vi "datalogger_all_signals_v3.0.vi"() -> ()   [LabVIEW 2017]
uses:
  <vilib>/Utility/file.llb/Write Delimited Spreadsheet (string).vi
  <vilib>/NI/Modbus Library/API/Wrapper/Create TCP Master.vi
  <vilib>/NI/Modbus Library/API/Master/Modbus Master.lvclass
  <instrlib>/Agilent 34970/Agilent 34970.lvlib
  <vilib>/NI/Modbus Library/API/Wrapper/API Main.lvlib
panel:
  out "Time constant 2":i32
  out "Time constant":i32
  in  "Tab Control":T1(tab)
  out "Indicator":bool
  in  "Touch the button to refresh":bool
  in  "Power on/off":u16(ring) items=["Power off", "Powe on"]
  in  "Mode selector":u16(ring) items=["Conditioning", "Activation"]
  out "Mode status":string
  out "Controller output 3 (V)":u16[](array[numeric])
  out "Controller outpu 2 (V)":u16[](array[numeric])
  out "Controller output 1 (V)":u16[](array[numeric])
  in  "Stop test":bool
  out "Controller temperature (Cº)":dbl[](array[numeric])
  out "Coil tempe (Cº)":dbl[](array[numeric])
  out "PT100 temp (Cº)":ext[](array[numeric])
  out "sampling time (ms)":u32
  out "Power consuption (W)":dbl[](array[numeric]) format="%.2f"
  in  "Datalogger_current\nGPIB1":refnum<visa-resource-name>="GPIB0::9::INSTR"
  in  "Datalogger_all_signals\nGPIB0":refnum<visa-resource-name>="GPIB0::9::INSTR"
  in  "Test type":u16(ring) items=["Final", "INITIAL", "PASSIVE", "ACTIVE"]
  in  "Axis orientation":u16(ring) items=["+x", "-x", "+y", "-y", "+z", "-z", "Reference Test"]
  out "minutos":u32
  out "segundos":u32
  out "Heating resistor 1":cluster{dbl[], dbl[]}[](graph)
  out "Heating resistor 1  DC voltage (v)":dbl[](array[numeric]) format="%.6f"
  out "Termocouple out1":dbl[](array[numeric])
  out "Heating resistor 1 P out (W)":dbl[](array[numeric])
  out "Heat resistor 1 resistance":dbl[](array[numeric]) format="%.2f"
  out "Heating resistor 2  DC voltage (v)":dbl[](array[numeric]) format="%.6f"
  out "Heating resistor 2 P out (W)":dbl[](array[numeric])
  out "Termocouple out2":dbl[](array[numeric])
  out "Heating resistor 2":cluster{dbl[], dbl[]}[](graph)
  out "Heat resistor 2 resistance":dbl[](array[numeric]) format="%.2f"
  out "Heating resistor 3  DC voltage (v)":dbl[](array[numeric]) format="%.6f"
  out "Heating resistor 3 P out (W)":dbl[](array[numeric])
  out "Termocouple out3":dbl[](array[numeric])
  out "Heating resistor 3":cluster{dbl[], dbl[]}[](graph)
  out "Heat resistor 3 resistance":dbl[](array[numeric]) format="%.2f"
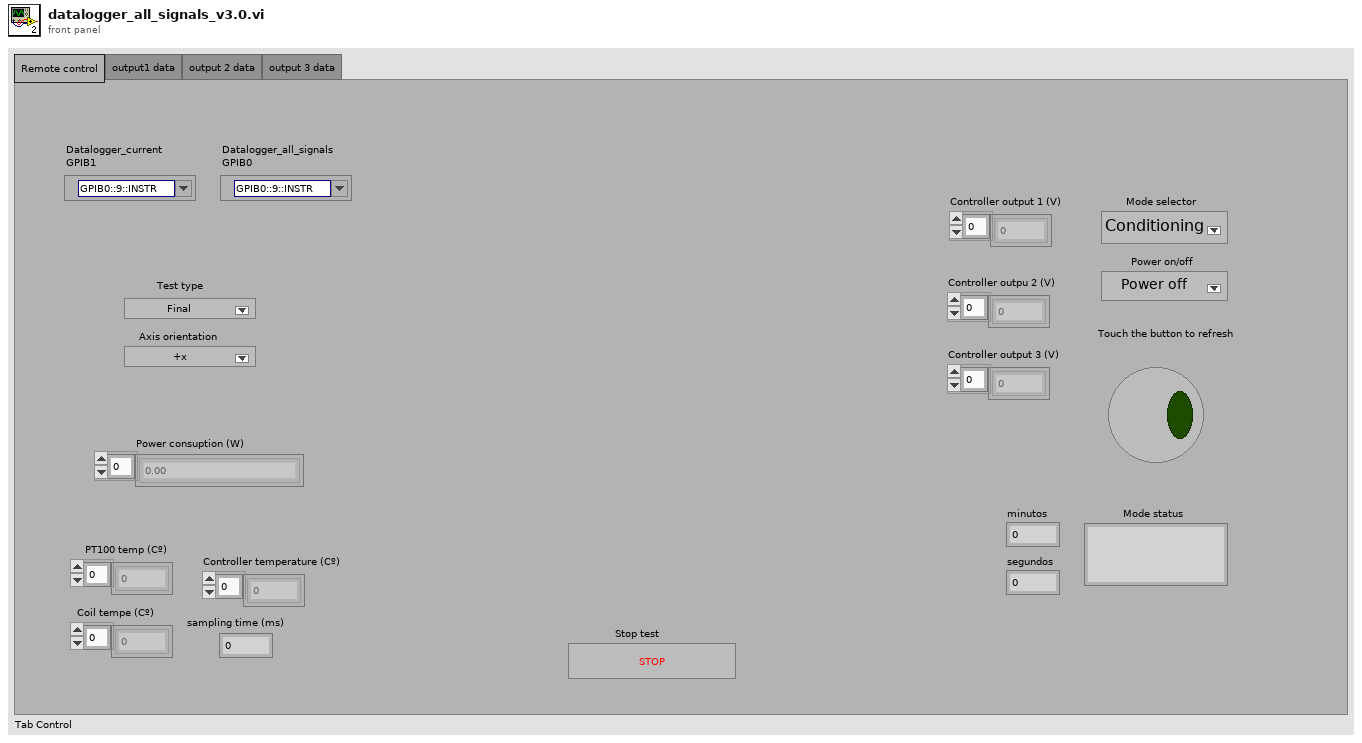
[diagram p1: front panel]
types:
  T1 = enum32{"Remote control", "output1 data", "output 2 data", "output 3 data"}
  T2 = enum16{"100 Ohm", "1 kOhm", "10 kOhm", "100 kOhm", "1 MOhm", "10 MOhm", "100 MOhm", "Auto", "Minimum", "Maximum"}
  T3 = enum16{"4 1/2", "5 1/2", "6 1/2", "Least", "Highest", "Default"}
  T4 = enum16{"100 mV", "1 V", "10 V", "100 V", "300 V", "Auto", "Minimum", "Maximum"}
  T5 = enum16{"B", "E", "J", "K", "N", "R", "S", "T", "Default (Last)"}
  T6 = enum16{"Thermocouple", "Thermistor", "RTD", "4-Wire RTD", "Default (Last)"}
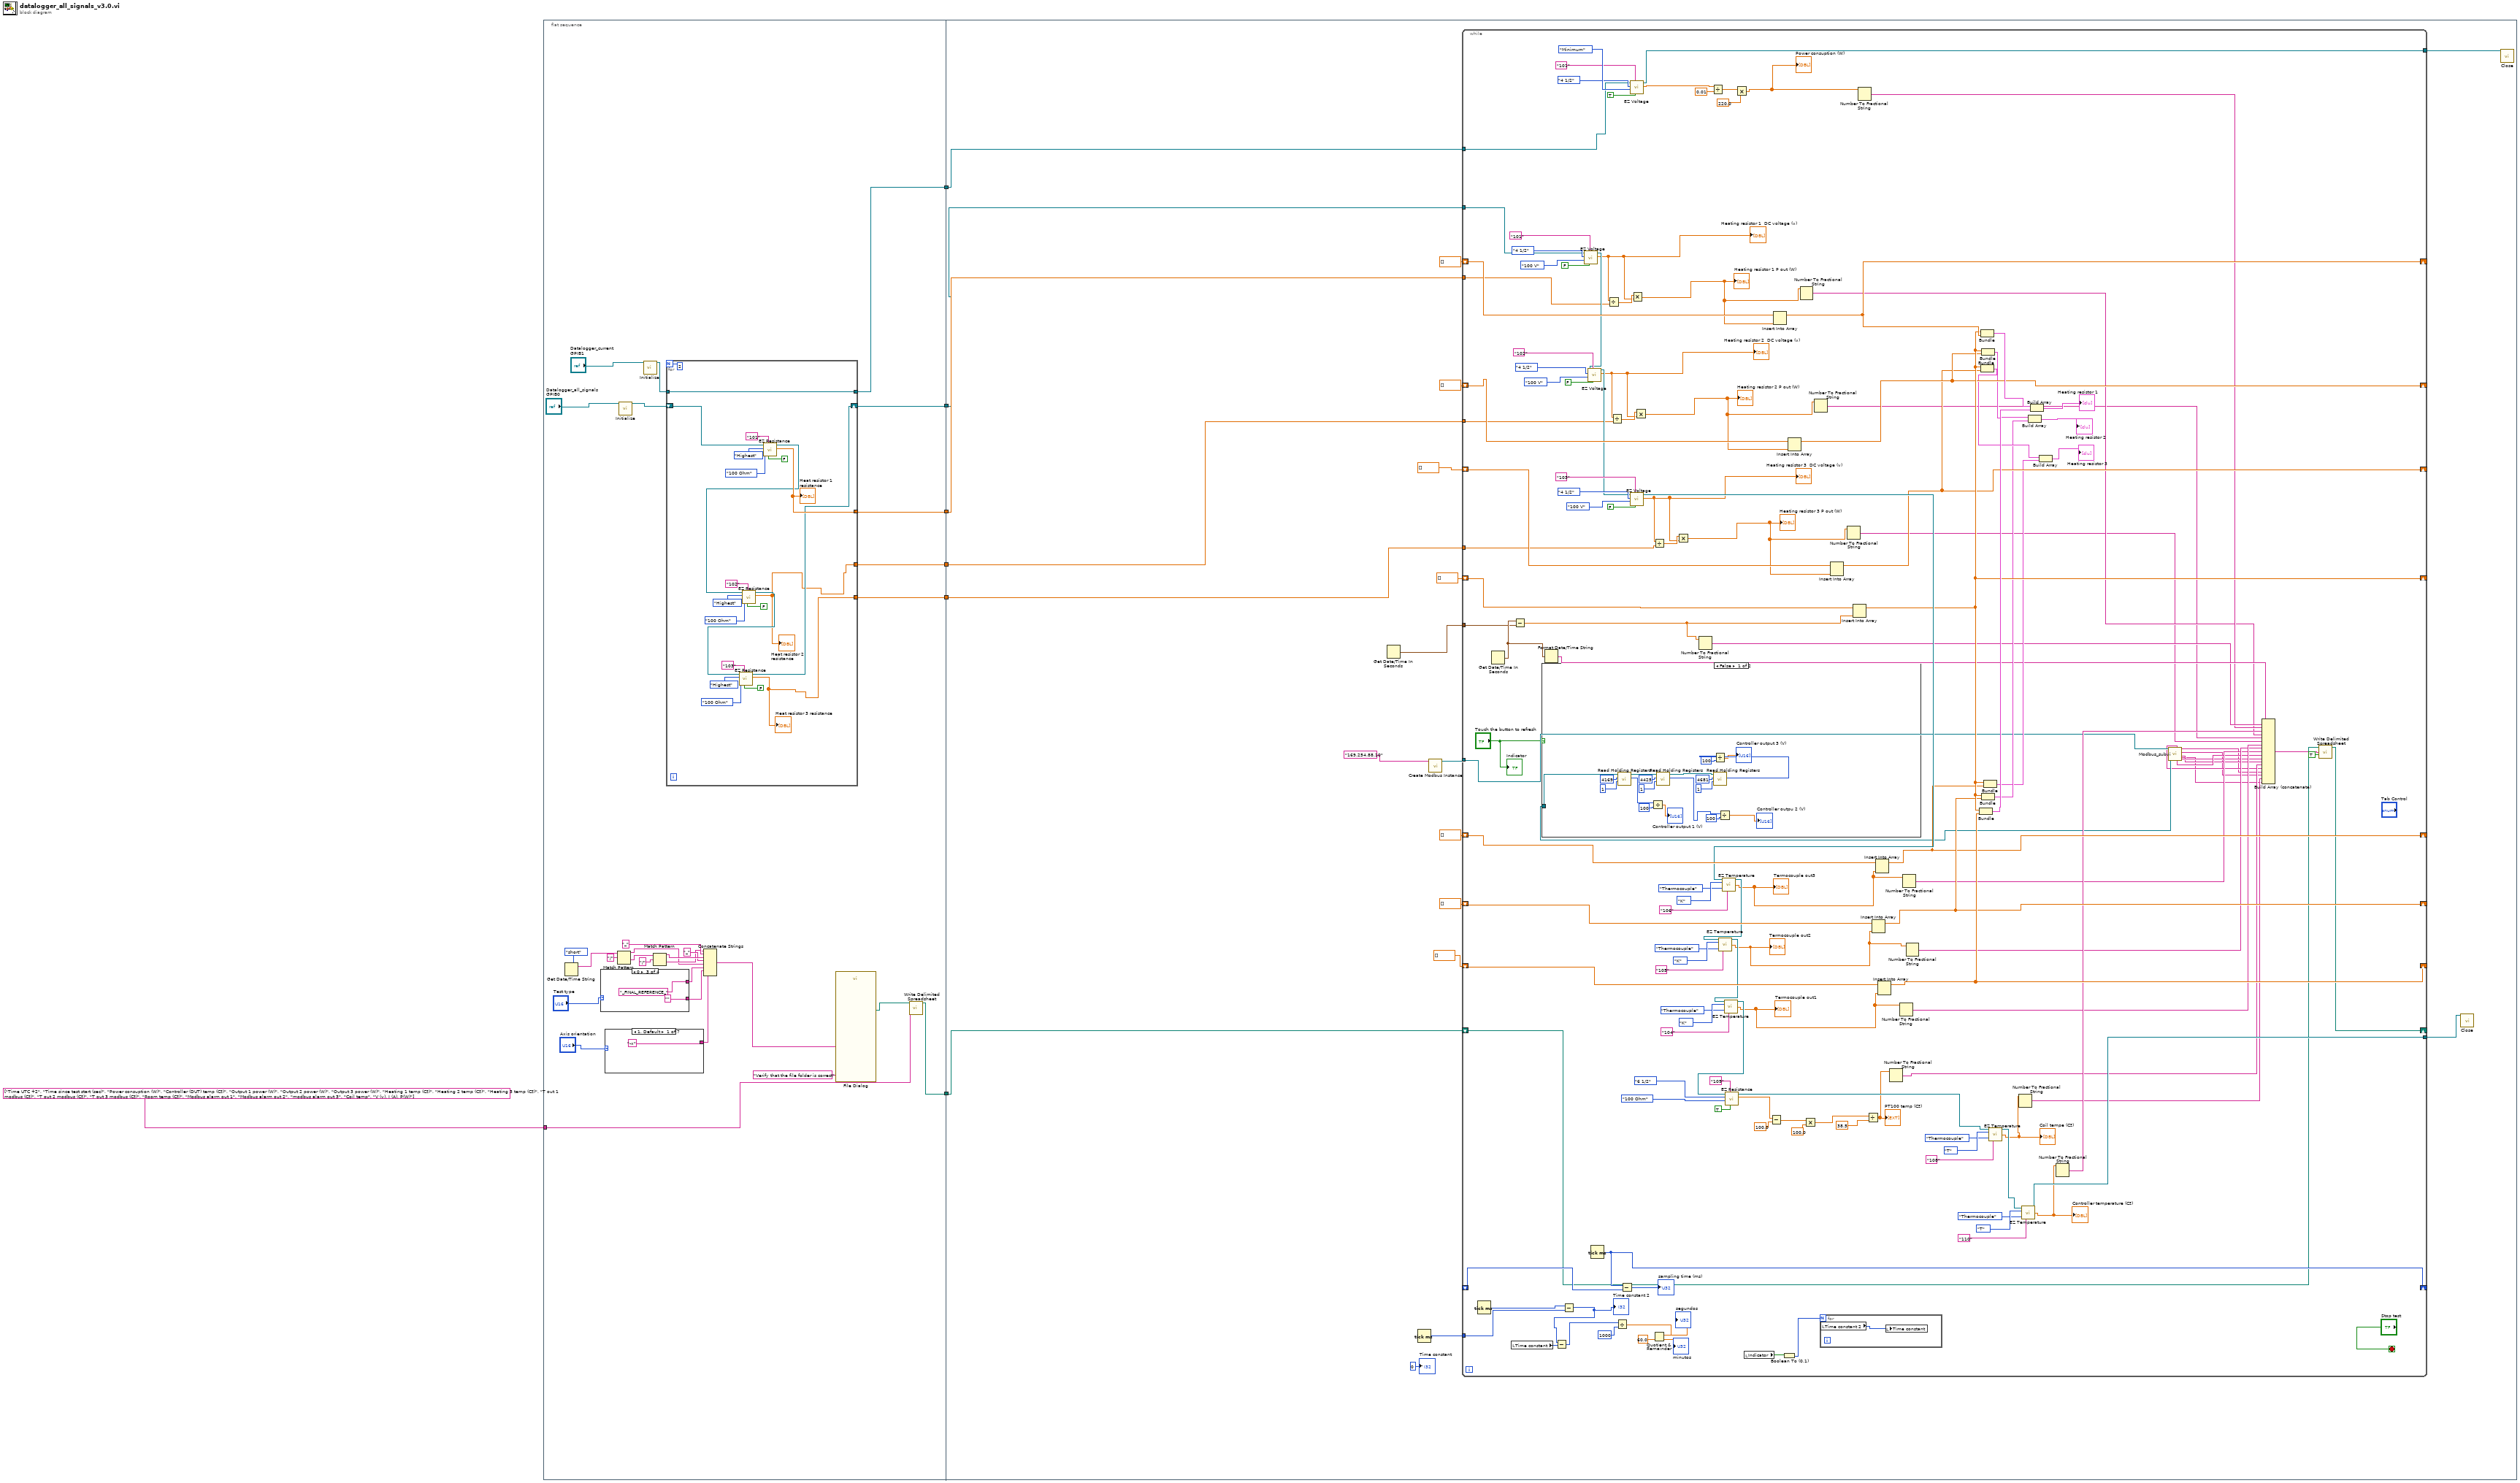
[diagram p0: block diagram]
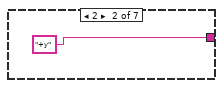
[diagram p2: hidden frame]
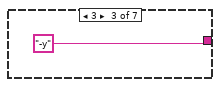
[diagram p3: hidden frame]
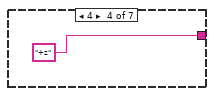
[diagram p4: hidden frame]
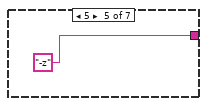
[diagram p5: hidden frame]
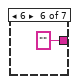
[diagram p6: hidden frame]
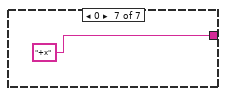
[diagram p7: hidden frame]
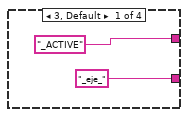
[diagram p8: hidden frame]
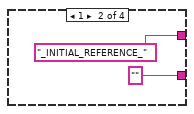
[diagram p9: hidden frame]
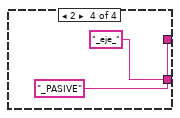
[diagram p10: hidden frame]
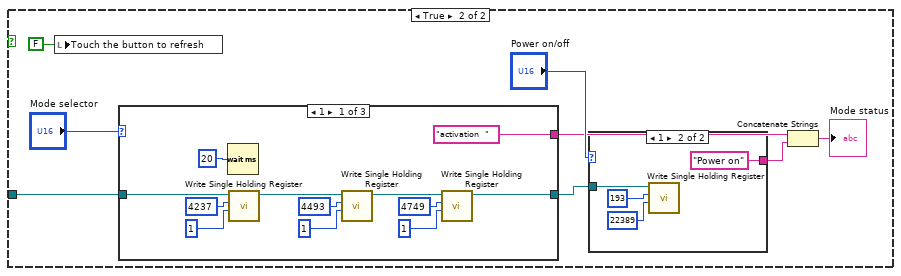
[diagram p11: hidden frame]
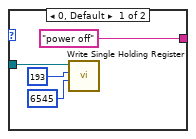
[diagram p12: hidden frame]
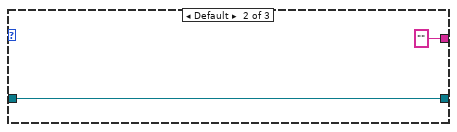
[diagram p13: hidden frame]
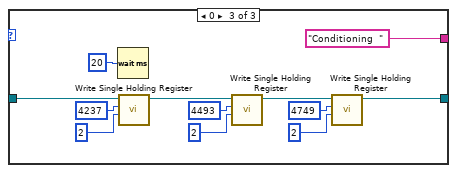
[diagram p14: hidden frame]
diagram:
  n1 = flat-sequence {
    tunnel: string[] ["Time UTC +2", "Time since test start (sec)", "Power consuption (W)", "Controller (DUT) temp (Cº)", "Output 1 power (W)", "Output 2 power (W)", "Output 3 power (W)", "Heating 1 temp (Cº)", "Heating 2 temp (Cº)", "Heating 3 temp (Cº)", "T out 1 modbus (Cº)", "T out 2 modbus (Cº)", "T out 3 modbus (Cº)", "Room temp (Cº)", "Modbus alarm out 1", "Modbus alarm out 2", "modbus alarm out 3", "Coil temp", "V (v), I (A), P(W)"] ("element") -> [w30]
    tunnel: [w34] -> w6
    tunnel: [w33] -> w5
    tunnel: [w32] -> w4
    tunnel: [w29] -> w3
    tunnel: [w28] -> w2
    tunnel: [w25] -> w1
    tunnel: w6 -> [w89]
    tunnel: w5 -> [w82]
    tunnel: w4 -> [w81]
    tunnel: w3 -> [w80]
    tunnel: w2 -> [w79]
    tunnel: w1 -> [w78]
    frame #0 {
      n2 = Get Date/Time String(date format (0)=enum16{"short", "long", "abbreviated"}."short") -> (date string=w19:string)  [unwired: 2 in, 1 out]
      n3 = case shown="0" "Test type" {
        tunnel: ["_ACTIVE" "_INITIAL_REFERENCE_" "_FINAL_REFERENCE_" "_PASIVE"] -> w23
        tunnel: ["_eje_" ("string") "" ("string") "" ("string") "_eje_" ("string")] -> w12
        frame 3, Default {
        }
        frame 1 {
        }
        frame 0 {
        }
        frame 2 {
        }
      }
      n4 = case shown="1, Default" "Axis orientation" {
        tunnel: ["-x" "+y" "-y" "+z" "-z" "" "+x"] -> w20
        frame 1, Default {
        }
        frame 2 {
        }
        frame 3 {
        }
        frame 4 {
        }
        frame 5 {
        }
        frame 6 {
        }
        frame 0 {
        }
      }
      n5 = Match Pattern(string=w19, regular expression="/") -> (before substring=w9:string, after substring=w16:string)  [unwired: 1 in, 2 out]
      n6 = call <instrlib>:"Initialize.vi"("VISA Resource Name"="Datalogger_all_signals\nGPIB0") -> ("VISA Resource Name Out"=w36:refnum<visa-resource-name>)  [unwired: 13 in, 1 out]
      n7 = call <instrlib>:"Initialize.vi"("VISA Resource Name"="Datalogger_current\nGPIB1") -> ("VISA Resource Name Out"=w26:refnum<visa-resource-name>)  [unwired: 13 in, 1 out]
      n8 = Match Pattern(string=w16, regular expression="/") -> (before substring=w14:string, after substring=w11:string)  [unwired: 1 in, 2 out]
      n9 = for {
        N: 2 -> [_]
        tunnel: [w67] -> w34
        shift-right: [w56] -> w28
        shift-left: w36 -> [w69]
        tunnel: [w55] -> w33
        tunnel: [w54] -> w32
        tunnel: w26 -> [w53]
        tunnel: [w53] -> w25
        n10 = call <instrlib>:"EZ Resistance.vi"("2w/4w (F:2w)"=FALSE, "Scan List (empty)"="101", "Range (7:Auto)"=T2."100 Ohm", "Resolution (5:Default)"=T3."Highest", "VISA Resource Name"=w69) -> ("Output Array"=w67:dbl[], "VISA Resource Name Out"=w58:refnum<visa-resource-name>)  [unwired: 4 in, 1 out]
        "Heat resistor 1 resistance" <- w67
        n11 = call <instrlib>:"EZ Resistance.vi"("2w/4w (F:2w)"=FALSE, "Scan List (empty)"="102", "Range (7:Auto)"=T2."100 Ohm", "Resolution (5:Default)"=T3."Highest", "VISA Resource Name"=w58) -> ("Output Array"=w55:dbl[], "VISA Resource Name Out"=w57:refnum<visa-resource-name>)  [unwired: 4 in, 1 out]
        "Heat resistor 2 resistance" <- w55
        n12 = call <instrlib>:"EZ Resistance.vi"("2w/4w (F:2w)"=FALSE, "Scan List (empty)"="103", "Range (7:Auto)"=T2."100 Ohm", "Resolution (5:Default)"=T3."Highest", "VISA Resource Name"=w57) -> ("Output Array"=w54:dbl[], "VISA Resource Name Out"=w56:refnum<visa-resource-name>)  [unwired: 4 in, 1 out]
        "Heat resistor 3 resistance" <- w54
      }
      n13 = Concatenate Strings(w11, "_" ("string"), w14, "_" ("string"), w9, w23, w12, w20) -> (w10:string)
      n14 = call "File Dialog"("prompt"="Verify that the file folder is correct", "default name"=w10) -> ("selected path"=w31:path)  [unwired: 10 in, 3 out]
      n15 = call-poly <vilib>:"Write Delimited Spreadsheet.vi"("file path (dialog if empty)"=w31, "1D data"=w30) -> ("new file path (Not A Path if cancelled)"=w29:path)  [unwired: 12 in, 1 out]
    }
    frame #1 {
      n16 = Get Date/Time In Seconds() -> (seconds since 1Jan1904=w75:timestamp)
      n17 = Tick Count (ms)() -> (millisecond timer value=w74:u32)
      n18 = call-poly <vilib>:"Create Modbus Instance.vi"("address"="169.254.88.10") -> ("TCP master instance"=w92:refnum<class "Modbus Master.lvclass">)  [unwired: 9 in, 1 out]
      n19 = while {
        shift-right: [w231] -> _
        shift-left: _ -> [w230]
        tunnel: w89 -> [w175]
        shift-right: [w206] -> _
        shift-left: dbl[] [] -> [w208]
        shift-right: [w174] -> _
        shift-left: dbl[] [] -> [w207]
        shift-right: [w203] -> _
        shift-left: dbl[] [] -> [w205]
        shift-right: [w171] -> _
        shift-left: dbl[] [] -> [w195]
        shift-right: [w166] -> _
        shift-left: dbl[] [] -> [w189]
        shift-right: [w173] -> _
        shift-left: dbl[] [] -> [w185]
        shift-right: [w172] -> _
        shift-left: dbl[] [] -> [w180]
        tunnel: [w155] -> w90
        tunnel: w82 -> [w154]
        tunnel: w81 -> [w153]
        shift-right: [w137] -> _
        shift-left: w80 -> [w138]
        tunnel: w79 -> [w134]
        tunnel: [w133] -> w91
        tunnel: w78 -> [w132]
        tunnel: w92 -> [w118]
        tunnel: w75 -> [w108]
        tunnel: w74 -> [w100]
        stop <- "Stop test" stop-if-true
        n20 = Tick Count (ms)() -> (millisecond timer value=w101:u32)
        n21 = Get Date/Time In Seconds() -> (seconds since 1Jan1904=w152:timestamp)
        n22 = local read "Time constant"() -> (w99:i32)
        n23 = Subtract(x=w152, y=w108) -> (x-y=w128:dbl)
        n24 = Format Date/Time String(seconds (now)=w152) -> (date/time string=w151:string)  [unwired: 2 in]
        n25 = Subtract(x=w101, y=w100) -> (x-y=w94:u32)
        "Time constant 2" <- w94
        n26 = Subtract(x=w94, y=w99) -> (x-y=w98:u32)
        n27 = call <instrlib>:"EZ Voltage.vi"("AC/DC (F:DC)"=FALSE, "Scan List (empty)"="101", "Range (5:Auto)"=T4."100 V", "Resolution (5:Default)"=T3."4 1/2", "VISA Resource Name"=w134) -> ("Output Array"=w150:dbl[], "VISA Resource Name Out"=w178:refnum<visa-resource-name>)  [unwired: 4 in, 1 out]
        "Heating resistor 1  DC voltage (v)" <- w150
        n28 = call <instrlib>:"EZ Voltage.vi"("AC/DC (F:DC)"=FALSE, "Scan List (empty)"="102", "Range (5:Auto)"=T4."100 V", "Resolution (5:Default)"=T3."4 1/2", "VISA Resource Name"=w178) -> ("Output Array"=w148:dbl[], "VISA Resource Name Out"=w177:refnum<visa-resource-name>)  [unwired: 4 in, 1 out]
        "Heating resistor 2  DC voltage (v)" <- w148
        n29 = Tick Count (ms)() -> (millisecond timer value=w231:u32)
        n30 = Divide(x=w150, y=w175) -> (x/y=w209:dbl[])
        n31 = Divide(x=w148, y=w154) -> (x/y=w196:dbl[])
        n32 = Divide(x=w98, y=u32 1000) -> (x/y=w104:dbl)
        n33 = Subtract(x=w231, y=w230) -> (x-y=→"sampling time (ms)":u32)
        n34 = call <instrlib>:"EZ Voltage.vi"("AC/DC (F:DC)"=TRUE, "Scan List (empty)"="101", "Range (5:Auto)"=T4."Minimum", "Resolution (5:Default)"=T3."4 1/2", "VISA Resource Name"=w132) -> ("Output Array"=w232:dbl[], "VISA Resource Name Out"=w133:refnum<visa-resource-name>)  [unwired: 4 in, 1 out]
        n35 = call <instrlib>:"EZ Voltage.vi"("AC/DC (F:DC)"=FALSE, "Scan List (empty)"="103", "Range (5:Auto)"=T4."100 V", "Resolution (5:Default)"=T3."4 1/2", "VISA Resource Name"=w177) -> ("Output Array"=w146:dbl[], "VISA Resource Name Out"=w176:refnum<visa-resource-name>)  [unwired: 4 in, 1 out]
        "Heating resistor 3  DC voltage (v)" <- w146
        n36 = Multiply(x=w209, y=w150) -> (x*y=w149:dbl[])
        "Heating resistor 1 P out (W)" <- w149
        n37 = Multiply(x=w196, y=w148) -> (x*y=w147:dbl[])
        "Heating resistor 2 P out (W)" <- w147
        n38 = Quotient & Remainder(x=w104, y=60.0) -> (x-y*floor(x/y)=→"segundos":dbl, floor(x/y)=→"minutos":dbl)
        n39 = Divide(x=w146, y=w153) -> (x/y=w190:dbl[])
        n40 = Multiply(x=w190, y=w146) -> (x*y=w145:dbl[])
        "Heating resistor 3 P out (W)" <- w145
        n41 = Number To Fractional String(number=w128) -> (F-format string=w127:string)  [unwired: 3 in]
        n42 = Divide(x=w232, y=0.01) -> (x/y=w131:dbl[])
        n43 = call <instrlib>:"EZ Temperature.vi"("VISA Resource Name"=w176, "Scan List (empty)"="106" ("Channel List"), "Thermocouple Type (8:Def-Last)"=T5."K", "Transducer Type (4:Def-Last)"=T6."Thermocouple") -> ("VISA Resource Name Out"=w179:refnum<visa-resource-name>, "Output Array"=w142:dbl[])  [unwired: 9 in, 1 out]
        "Termocouple out3" <- w142
        n44 = call <instrlib>:"EZ Temperature.vi"("VISA Resource Name"=w179, "Scan List (empty)"="105" ("Channel List"), "Thermocouple Type (8:Def-Last)"=T5."K", "Transducer Type (4:Def-Last)"=T6."Thermocouple") -> ("VISA Resource Name Out"=w184:refnum<visa-resource-name>, "Output Array"=w143:dbl[])  [unwired: 9 in, 1 out]
        "Termocouple out2" <- w143
        n45 = call <instrlib>:"EZ Temperature.vi"("VISA Resource Name"=w184, "Scan List (empty)"="104" ("Channel List"), "Thermocouple Type (8:Def-Last)"=T5."K", "Transducer Type (4:Def-Last)"=T6."Thermocouple") -> ("VISA Resource Name Out"=w210:refnum<visa-resource-name>, "Output Array"=w144:dbl[])  [unwired: 9 in, 1 out]
        "Termocouple out1" <- w144
        n46 = call <instrlib>:"EZ Resistance.vi"("2w/4w (F:2w)"=TRUE, "Scan List (empty)"="109", "Range (7:Auto)"=T2."100 Ohm", "Resolution (5:Default)"=T3."6 1/2", "VISA Resource Name"=w210) -> ("Output Array"=w213:dbl[], "VISA Resource Name Out"=w160:refnum<visa-resource-name>)  [unwired: 4 in, 1 out]
        n47 = Multiply(x=w131, y=220.0) -> (x*y=w129:dbl[])
        "Power consuption (W)" <- w129
        n48 = local read "Indicator"() -> (w96:bool)
        n49 = Subtract(x=w213, y=100.0) -> (x-y=w211:dbl[])
        n50 = Insert Into Array(array=w205, new element=w149) -> (w203:dbl[])  [unwired: 1 in]
        n51 = Boolean To (0,1)(Boolean=w96) -> (0, 1=w95:i16)
        n52 = Insert Into Array(array=w195, new element=w147) -> (w171:dbl[])  [unwired: 1 in]
        n53 = Number To Fractional String(number=w149) -> (F-format string=w124:string[])  [unwired: 3 in]
        n54 = Multiply(x=w211, y=100.0) -> (x*y=w215:ext[])
        n55 = Number To Fractional String(number=w147) -> (F-format string=w123:string[])  [unwired: 3 in]
        n56 = for {
          N: w95 -> [_]
          n57 = local read "Time constant 2"() -> (w237:i32)
          n58 = local write "Time constant"(w237) -> ()
        }
        n59 = Insert Into Array(array=w189, new element=w145) -> (w166:dbl[])  [unwired: 1 in]
        n60 = Number To Fractional String(number=w145) -> (F-format string=w122:string[])  [unwired: 3 in]
        n61 = Insert Into Array(array=w207, new element=w128) -> (w174:dbl[])  [unwired: 1 in]
        n62 = Number To Fractional String(number=w129) -> (F-format string=w126:string[])  [unwired: 3 in]
        n63 = Divide(x=w215, y=38.5) -> (x/y=w141:ext[])
        "PT100 temp (Cº)" <- w141
        n64 = Insert Into Array(array=w185, new element=w143) -> (w173:dbl[])  [unwired: 1 in]
        n65 = Insert Into Array(array=w180, new element=w142) -> (w172:dbl[])  [unwired: 1 in]
        n66 = Insert Into Array(array=w208, new element=w144) -> (w206:dbl[])  [unwired: 1 in]
        n67 = Number To Fractional String(number=w141) -> (F-format string=w113:string[])  [unwired: 3 in]
        n68 = Number To Fractional String(number=w144) -> (F-format string=w121:string[])  [unwired: 3 in]
        n69 = Number To Fractional String(number=w142) -> (F-format string=w119:string[])  [unwired: 3 in]
        n70 = Number To Fractional String(number=w143) -> (F-format string=w120:string[])  [unwired: 3 in]
        n71 = Bundle(w174, w206) -> (w204:cluster{dbl[], dbl[]})  [unwired: 1 in]
        n72 = Bundle(w174, w203) -> (w202:cluster{dbl[], dbl[]})  [unwired: 1 in]
        n73 = Bundle(w174, w166) -> (w167:cluster{dbl[], dbl[]})  [unwired: 1 in]
        n74 = Bundle(w174, w171) -> (w168:cluster{dbl[], dbl[]})  [unwired: 1 in]
        n75 = Bundle(w174, w173) -> (w165:cluster{dbl[], dbl[]})  [unwired: 1 in]
        n76 = Bundle(w174, w172) -> (w164:cluster{dbl[], dbl[]})  [unwired: 1 in]
        n77 = call <instrlib>:"EZ Temperature.vi"("VISA Resource Name"=w160, "Scan List (empty)"="108" ("Channel List"), "Thermocouple Type (8:Def-Last)"=T5."T", "Transducer Type (4:Def-Last)"=T6."Thermocouple") -> ("VISA Resource Name Out"=w156:refnum<visa-resource-name>, "Output Array"=w140:dbl[])  [unwired: 9 in, 1 out]
        "Coil tempe (Cº)" <- w140
        n78 = Number To Fractional String(number=w140) -> (F-format string=w109:string[])  [unwired: 3 in]
        n79 = call <instrlib>:"EZ Temperature.vi"("VISA Resource Name"=w156, "Scan List (empty)"="110" ("Channel List"), "Thermocouple Type (8:Def-Last)"=T5."T", "Transducer Type (4:Def-Last)"=T6."Thermocouple") -> ("VISA Resource Name Out"=w155:refnum<visa-resource-name>, "Output Array"=w139:dbl[])  [unwired: 9 in, 1 out]
        "Controller temperature (Cº)" <- w139
        n80 = Build Array(w168, w165) -> (→"Heating resistor 2":cluster{dbl[], dbl[]}[])
        n81 = Build Array(w202, w204) -> (→"Heating resistor 1":cluster{dbl[], dbl[]}[])
        n82 = Build Array(w167, w164) -> (→"Heating resistor 3":cluster{dbl[], dbl[]}[])
        n83 = Number To Fractional String(number=w139) -> (F-format string=w125:string[])  [unwired: 3 in]
        n84 = call "Modbus_subvi.vi"("Modbus master in"=w118) -> ("Output 2 temp alarm"=w115:string, "Output 3 temp alarm"=w114:string, "Controller output 3 alarm"=w110:string, "Controller output 2 alarm"=w111:string, "Output 1 temp alarm"=w116:string, "Controller output 1 alarm"=w112:string, "Variables voltage"=w93:string, "Modbus master out"=w117:refnum<class "Modbus Master.lvclass">)  [unwired: 3 in]
        n85 = case shown="False" "Touch the button to refresh" {
          tunnel: w117 -> [w253 w256]
          frame False {
            n86 = call-dynamic "Read Holding Registers.vi"("number of inputs"=u16 1, "starting address"=u32 4169, "Modbus master in"=w253) -> ("register values"=w246:u16[], "Modbus master out"=w248:refnum<class "Modbus Master.lvclass">)  [unwired: 6 in, 1 out]
            n87 = Divide(x=w246, y=u16 100) -> (x/y=→"Controller output 1 (V)":dbl[])
            n88 = call-dynamic "Read Holding Registers.vi"("number of inputs"=u16 1, "starting address"=u32 4425, "Modbus master in"=w248) -> ("register values"=w241:u16[], "Modbus master out"=w247:refnum<class "Modbus Master.lvclass">)  [unwired: 6 in, 1 out]
            n89 = call-dynamic "Read Holding Registers.vi"("number of inputs"=u16 1, "starting address"=u32 4681, "Modbus master in"=w247) -> ("register values"=w240:u16[])  [unwired: 6 in, 2 out]
            n90 = Divide(x=w240, y=u16 100) -> (x/y=→"Controller output 3 (V)":dbl[])
            n91 = Divide(x=w241, y=u16 100) -> (x/y=→"Controller outpu 2 (V)":dbl[])
          }
          frame True {
            n92 = local write "Touch the button to refresh"(FALSE ("Boolean")) -> ()
            n93 = case shown="1" "Mode selector" {
              tunnel: w256 -> [w275 w285 w289]
              tunnel: [w274 w285 w288] -> w262
              tunnel: ["activation  " ("Mode") "" ("Mode") "Conditioning  " ("Mode")] -> w259
              frame 1 {
                n94 = Wait (ms)(milliseconds to wait=u32 20) -> ()  [unwired: 1 out]
                n95 = call-dynamic "Write Single Holding Register.vi"("register to write"=u16 1 ("register to write 2"), "address"=u16 4237, "Modbus master in"=w275) -> ("Modbus master out"=w277:refnum<class "Modbus Master.lvclass">)  [unwired: 7 in, 1 out]
                n96 = call-dynamic "Write Single Holding Register.vi"("register to write"=u16 1 ("register to write 2"), "address"=u16 4493, "Modbus master in"=w277) -> ("Modbus master out"=w276:refnum<class "Modbus Master.lvclass">)  [unwired: 7 in, 1 out]
                n97 = call-dynamic "Write Single Holding Register.vi"("register to write"=u16 1 ("register to write 2"), "address"=u16 4749, "Modbus master in"=w276) -> ("Modbus master out"=w274:refnum<class "Modbus Master.lvclass">)  [unwired: 7 in, 1 out]
              }
              frame Default {
              }
              frame 0 {
                n98 = Wait (ms)(milliseconds to wait=u32 20) -> ()  [unwired: 1 out]
                n99 = call-dynamic "Write Single Holding Register.vi"("register to write"=u16 2 ("register to write 2"), "address"=u16 4237, "Modbus master in"=w289) -> ("Modbus master out"=w291:refnum<class "Modbus Master.lvclass">)  [unwired: 7 in, 1 out]
                n100 = call-dynamic "Write Single Holding Register.vi"("register to write"=u16 2 ("register to write 2"), "address"=u16 4493, "Modbus master in"=w291) -> ("Modbus master out"=w290:refnum<class "Modbus Master.lvclass">)  [unwired: 7 in, 1 out]
                n101 = call-dynamic "Write Single Holding Register.vi"("register to write"=u16 2 ("register to write 2"), "address"=u16 4749, "Modbus master in"=w290) -> ("Modbus master out"=w288:refnum<class "Modbus Master.lvclass">)  [unwired: 7 in, 1 out]
              }
            }
            n102 = case shown="1" "Power on/off" {
              tunnel: w262 -> [w265 w270]
              tunnel: ["power off" ("Mode") "Power on" ("Mode")] -> w258
              frame 0, Default {
                n103 = call-dynamic "Write Single Holding Register.vi"("register to write"=u16 6545, "address"=u16 193, "Modbus master in"=w265) -> ()  [unwired: 7 in, 2 out]
              }
              frame 1 {
                n104 = call-dynamic "Write Single Holding Register.vi"("register to write"=u16 22389, "address"=u16 193, "Modbus master in"=w270) -> ()  [unwired: 7 in, 2 out]
              }
            }
            n105 = Concatenate Strings(w259, w258) -> (→"Mode status":string)
          }
        }
        n106 = Build Array (concatenate)(w151, w127, w126, w125, w124, w123, w122, w121, w120, w119, w116, w115, w114, w113, w112, w111, w110, w109, w93) -> (w135:string[])
        n107 = call-poly <vilib>:"Write Delimited Spreadsheet.vi"("file path (dialog if empty)"=w138, "1D data"=w135, "append to file? (new file:F)"=TRUE) -> ("new file path (Not A Path if cancelled)"=w137:path)  [unwired: 11 in, 1 out]
        "Indicator" <- "Touch the button to refresh"
      }
      n108 = call <instrlib>:"Close.vi"("VISA Resource Name"=w90) -> ()  [unwired: 14 in, 1 out]
      n109 = call <instrlib>:"Close.vi"("VISA Resource Name"=w91) -> ()  [unwired: 14 in, 1 out]
      "Time constant" <- 0 ("Constant")
    }
  }
